vi "Read.vi"(8 "error in (no error)":errorcluster, 9 "Starting independent variable":dbl, 10 "Current independent variable":dbl, 11 "Reader in":refnum<class "Reader.lvclass">) -> (0 "error out":errorcluster, 2 "Data Channels":T1, 3 "Reader out":refnum<class "Reader.lvclass">)   [LabVIEW 2009, in "Reader.lvclass"]
doc: "Prepare for read, wait the time delay, and take data from up to 4 channels."
uses:
  Reader.lvclass
  Instruments/Utility Classes/Readable/Data Channels.ctl
  Instruments/Utility Classes/Readable/Data Channel.ctl
  Instruments/Utility Classes/Readable/Data Point.ctl
  Reader.lvclass/Reader.ctl
  Instruments/Utility Classes/Readable/Readable.lvclass
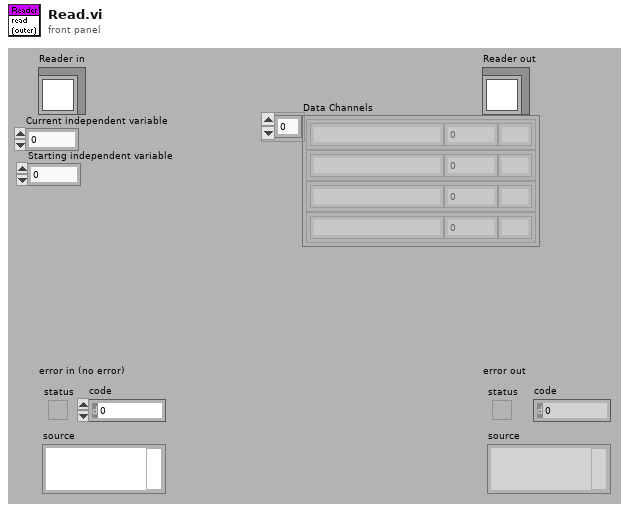
[diagram p1: front panel]
types:
  T1 = typedef "Readable.lvclass/Data Channels.ctl" = T2[]
  T2 = typedef "Readable.lvclass/Data Channel.ctl" = cluster{"Name":string, "Data Point":T3, "Unit":string}
  T3 = typedef "Readable.lvclass/Data Point.ctl" = dbl
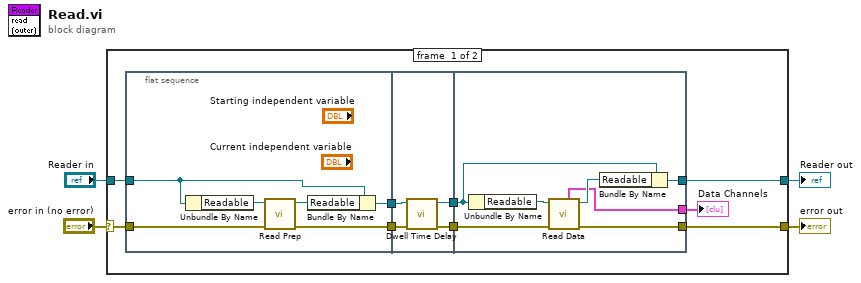
[diagram p0: block diagram]
diagram:
  n1 = case shown="No Error" "error in (no error)" {
    selector: "error in (no error)" -> [w11 w32]
    tunnel: [w10 w32] -> w3
    tunnel: [w5 w31] -> w1
    tunnel: "Reader in" -> [w6 w31]
    frame #0 {
      n2 = flat-sequence {
        tunnel: [w19] -> w13
        tunnel: w11 -> [w18]
        tunnel: w6 -> [w15]
        tunnel: [w16] -> w8
        tunnel: w13 -> [w23]
        tunnel: [w22] -> w12
        tunnel: w8 -> [w21]
        tunnel: [w20] -> w7
        tunnel: [w30] -> w10
        tunnel: w12 -> [w29]
        tunnel: [w24] -> w9
        tunnel: w7 -> [w25]
        tunnel: [w27] -> w5
        frame #0 {
          n3 = Unbundle By Name(w15) -> ("Readable"=w14:refnum<class "Readable.lvclass">)
          n4 = call-dynamic "Read Prep.vi"("error in (no error)"=w18, "Readable in"=w14) -> ("error out"=w19:errorcluster, "Readable out"=w17:refnum<class "Readable.lvclass">)  [unwired: 2 in, 6 out]
          n5 = Bundle By Name(cluster=w15, "Readable"=w17) -> (w16:refnum<class "Reader.lvclass">)
        }
        frame #1 {
          n6 = call-dynamic "Dwell Time Delay.vi"("error in (no error)"=w23, "Reader in"=w21) -> ("error out"=w22:errorcluster, "Reader out"=w20:refnum<class "Reader.lvclass">)  [unwired: 8 out]
        }
        frame #2 {
          n7 = Unbundle By Name(w25) -> ("Readable"=w28:refnum<class "Readable.lvclass">)
          n8 = call "Read Data.vi"("error in (no error)"=w29, "Readable in"=w28) -> ("error out"=w30:errorcluster, "Readable out"=w26:refnum<class "Readable.lvclass">, "Data Channels"=w24:T1)  [unwired: 7 out]
          n9 = Bundle By Name(cluster=w25, "Readable"=w26) -> (w27:refnum<class "Reader.lvclass">)
        }
      }
      "Data Channels" <- w9
    }
    frame #1 {
    }
  }
  "error out" <- w3
  "Reader out" <- w1
